vi "test - strip brackets.vi"() -> ()   [LabVIEW 2017]
panel:
  out "trimmed string out 2":string
  out "trimmed string out":string
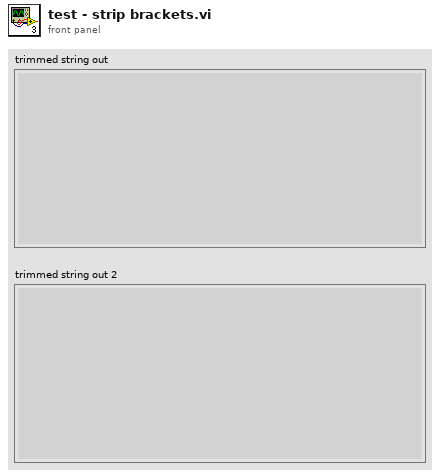
[diagram p1: front panel]
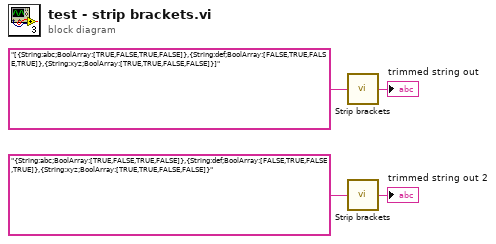
[diagram p0: block diagram]
diagram:
  n1 = call "Strip brackets.vi"("trimmed string in"="[{String:abc;BoolArray:[TRUE,FALSE,TRUE,FALSE]},{String:def;BoolArray:[FALSE,TRUE,FALSE,TRUE]},{String:xyz;BoolArray:[TRUE,TRUE,FALSE,FALSE]}]") -> ("trimmed string out"=→"trimmed string out":string)  [unwired: 3 in]
  n2 = call "Strip brackets.vi"("trimmed string in"="{String:abc;BoolArray:[TRUE,FALSE,TRUE,FALSE]},{String:def;BoolArray:[FALSE,TRUE,FALSE,TRUE]},{String:xyz;BoolArray:[TRUE,TRUE,FALSE,FALSE]}") -> ("trimmed string out"=→"trimmed string out 2":string)  [unwired: 3 in]
